vi "WSVCAP SHL Host LL RFFE Build and Parse Write Message.vi"(0 "Write Data In [DUT Ordered]":u8[][](array[numeric]) format="%02x", 1 "Message In":string, 5 "Socket Mask [U16] In":u16=1 format="%04x", 7 "Cycle CMD Lengths (bits)":u8[](array[numeric]), 9 "Cycle CMD Delay (ticks)":u32[](array[numeric]), 11 "error in":errorcluster) -> (3 "Message Out":string, 4 "Write Data Out [DUT Ordered]":u8[][](array[numeric]) format="%02x", 6 "Socket Mask [U16] Out":u16=1 format="%04x", 8 "Cycle CMD Lengths Out (bits)":u8[](array[numeric]), 10 "Cycle CMD Delay Out (ticks)":u32[](array[numeric]), 14 "Byte Count":u8, 15 "error out":errorcluster)   [LabVIEW 2012]
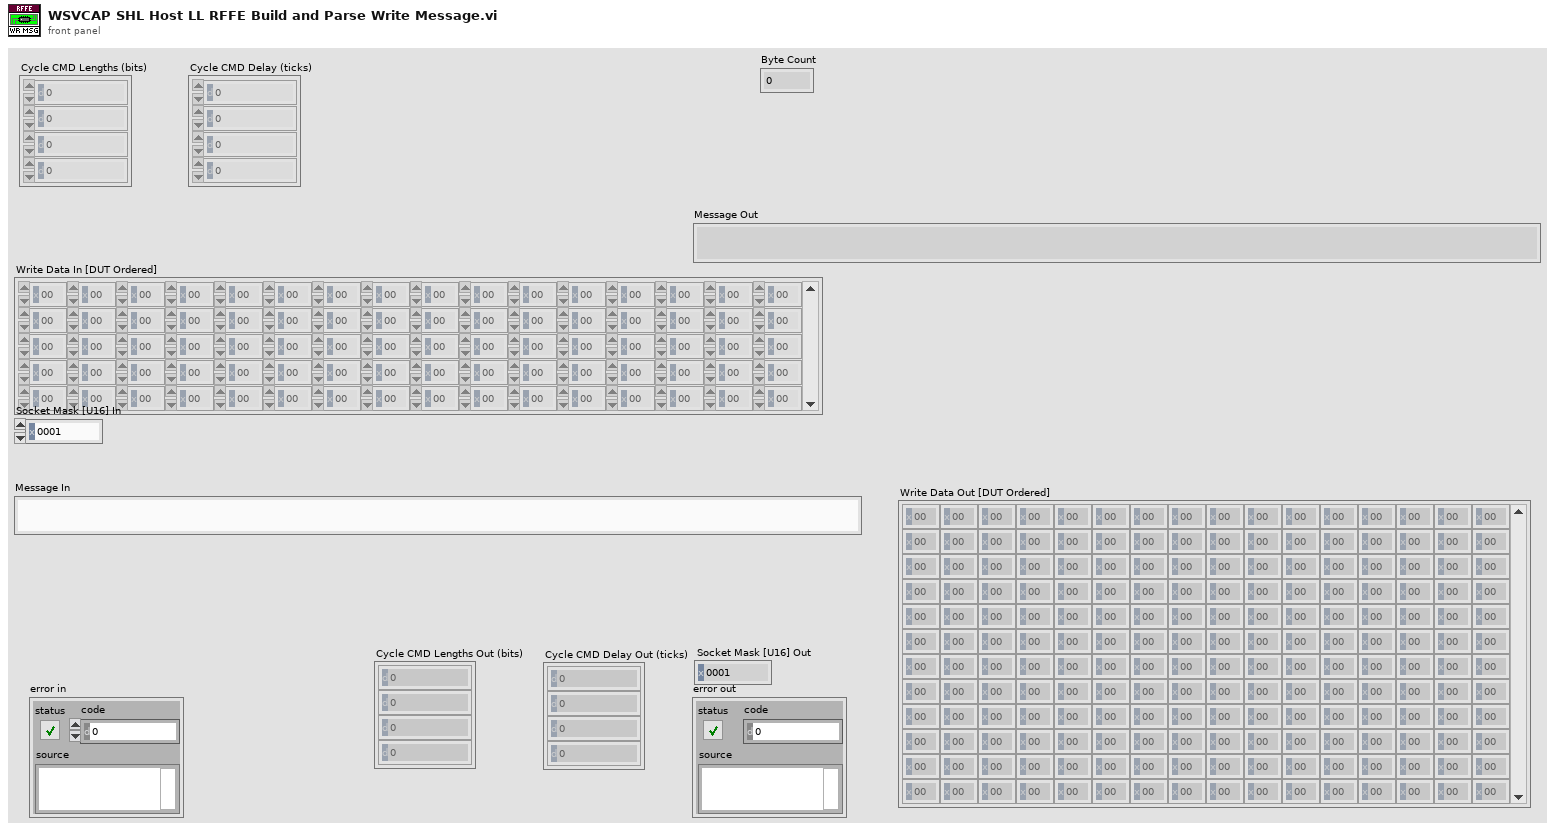
[diagram p1: front panel]
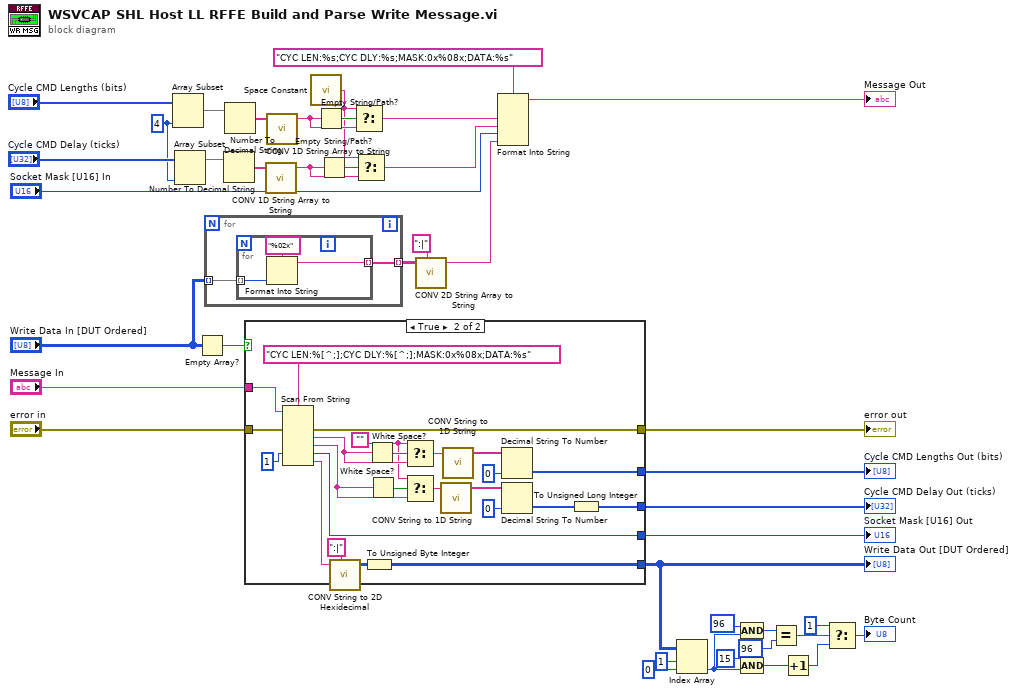
[diagram p0: block diagram]
diagram:
  w25 = 4 ("length")
  n1 = Array Subset(array="Cycle CMD Lengths (bits)", length=w25) -> (w28:u8[])  [unwired: 1 in]
  n2 = Array Subset(array="Cycle CMD Delay (ticks)", length=w25) -> (w26:u32[])  [unwired: 1 in]
  n3 = Empty Array?(array="Write Data In [DUT Ordered]") -> (empty?=w34:bool)
  n4 = for {
    tunnel: "Write Data In [DUT Ordered]" -> [w43] mode=indexing
    tunnel: [w42] -> w16 mode=indexing
    n5 = for {
      tunnel: w43 -> [w46] mode=indexing
      tunnel: [w45] -> w42 mode=indexing
      n6 = Format Into String(format string="%02x", w46) -> (resulting string=w45:string)  [unwired: 2 in, 1 out]
    }
  }
  n7 = Number To Decimal String(number=w26) -> (decimal integer string=w32:string[])  [unwired: 1 in]
  n8 = Number To Decimal String(number=w28) -> (decimal integer string=w33:string[])  [unwired: 1 in]
  n9 = case shown="True" w34 {
    tunnel: [_ w70] -> w10
    tunnel: [_ w68] -> w39
    tunnel: "error in" -> [w47 w66]
    tunnel: [w47 w65] -> w37
    tunnel: "Message In" -> [_ w63]
    tunnel: [_ w57] -> w31
    tunnel: [_ w48] -> w30
    frame False {
    }
    frame True {
      w49 = ""
      n10 = Scan From String(format string="CYC LEN:%[^;];CYC DLY:%[^;];MASK:0x%08x;DATA:%s", input string=w63, error in=w66, default 3=u16 1 ("Socket Mask [U16] Out")) -> (error out=w65:errorcluster, output 1=w52:string, output 2=w53:string, output 3=w68:u16, output 4=w67:string)  [unwired: 4 in, 2 out]
      n11 = call "CONV String to 2D Hexidecimal.vi"("String"=w67, "Delimiters (,;)"=":|") -> ("2-D Hexidecimal"=w71:u32[][])  [unwired: 7 in]
      n12 = To Unsigned Byte Integer(number=w71) -> (unsigned 8bit integer=w70:u8[][])
      n13 = White Space?(1:w52) -> (0:w51:bool)
      n14 = White Space?(1:w53) -> (0:w50:bool)
      n15 = Select(t=w49, s=w51, f=w52) -> (s? t:f=w55:string)
      n16 = Select(t=w49, s=w50, f=w53) -> (s? t:f=w54:string)
      n17 = call "CONV String to 1D String.vi"("String"=w54) -> ("1-D String"=w60:string[])  [unwired: 8 in]
      n18 = call "CONV String to 1D String.vi"("String"=w55) -> ("1-D String"=w61:string[])  [unwired: 8 in]
      n19 = Decimal String To Number(string=w61, default (0L)=u8 0 ("Read Data")) -> (number=w57:u8[])  [unwired: 1 in, 1 out]
      n20 = Decimal String To Number(string=w60, default (0L)=u64 0 ("Read Data")) -> (number=w56:u64[])  [unwired: 1 in, 1 out]
      n21 = To Unsigned Long Integer(number=w56) -> (unsigned 32bit integer=w48:u32[])
    }
  }
  "Write Data Out [DUT Ordered]" <- w10
  "Socket Mask [U16] Out" <- w39
  "error out" <- w37
  "Cycle CMD Lengths Out (bits)" <- w31
  "Cycle CMD Delay Out (ticks)" <- w30
  n22 = call "CONV 1D String Array to String.vi"("1-D String"=w32) -> ("String"=w21:string)  [unwired: 1 in, 7 out]
  n23 = call "CONV 1D String Array to String.vi"("1-D String"=w33) -> ("String"=w23:string)  [unwired: 1 in, 7 out]
  n24 = call <vilib>:"Space Constant.vi"() -> ("String"=w20:string)
  n25 = Empty String/Path?(string/path=w23) -> (empty?=w24:bool)
  n26 = Empty String/Path?(string/path=w21) -> (empty?=w22:bool)
  n27 = Select(t=w20, s=w24, f=w23) -> (s? t:f=w19:string)
  n28 = Select(t=w20, s=w22, f=w21) -> (s? t:f=w18:string)
  n29 = call "CONV 2D String Array to String.vi"("2-D String"=w16, "Delimiters (,;)"=":|") -> ("String"=w15:string)  [unwired: 7 in]
  n30 = Format Into String(format string="CYC LEN:%s;CYC DLY:%s;MASK:0x%08x;DATA:%s", w19, w18, "Socket Mask [U16] In", w15) -> (resulting string=→"Message Out":string)  [unwired: 2 in, 1 out]
  n31 = Index Array(array=w10, index (row)=1, index (col)=0 ("disabled index (col)")) -> (element=w7:u8)
  n32 = Compound Arithmetic op=AND(u8 96 ("index (row)"), w7) -> (w6:u8)
  n33 = Compound Arithmetic op=AND(u8 15 ("index (row)"), w7) -> (w11:u8)
  n34 = Equal?(x=w6, y=u8 96) -> (x = y?=w4:bool)
  n35 = Increment(x=w11) -> (x+1=w2:u8)
  n36 = Select(t=u8 1 ("Byte Count"), s=w4, f=w2) -> (s? t:f=→"Byte Count":u8)
